vi "7.0-Convert Tabs.vi"(1 "Tab Control":T1(ring)) -> (0 "7.0 GUI Tab Equivalent State":T2)   [LabVIEW 2010]
uses:
  7.0-OCU State.ctl
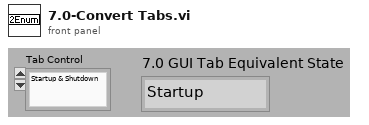
[diagram p1: front panel]
types:
  T1 = enum32{"Startup & Shutdown", "Self Test", "Manual Mode", "Auto Mode", "Mission Planning", "Timing"}
  T2 = typedef "7.0-OCU State.ctl" = enum16{"Startup", "Self Test", "Manual Mode", "Auto Mode", "Plan Mission", "Shutdown"}
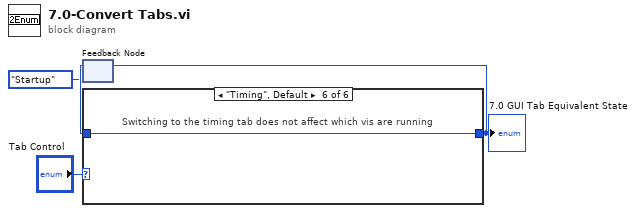
[diagram p0: block diagram]
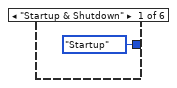
[diagram p2: hidden frame]
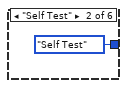
[diagram p3: hidden frame]
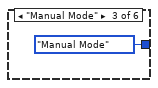
[diagram p4: hidden frame]
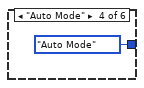
[diagram p5: hidden frame]
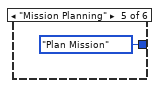
[diagram p6: hidden frame]
diagram:
  n1 = feedback #1(7.0-OCU_State."Startup" ("7.0 GUI Tab Equivalent State")) -> (w2:T2)
  n2 = case shown="\"Timing\", Default" "Tab Control" {
    tunnel: [7.0-OCU_State."Startup" ("7.0 GUI Tab Equivalent State") 7.0-OCU_State."Self Test" ("7.0 GUI Tab Equivalent State") 7.0-OCU_State."Manual Mode" ("7.0 GUI Tab Equivalent State") 7.0-OCU_State."Auto Mode" ("7.0 GUI Tab Equivalent State") 7.0-OCU_State."Plan Mission" ("7.0 GUI Tab Equivalent State") w10] -> w3
    tunnel: w2 -> [_ _ _ _ _ w10]
    frame "Startup & Shutdown" {
    }
    frame "Self Test" {
    }
    frame "Manual Mode" {
    }
    frame "Auto Mode" {
    }
    frame "Mission Planning" {
    }
    frame "Timing", Default {
      # "Switching to the timing tab does not affect which vis are running"
    }
  }
  "7.0 GUI Tab Equivalent State" <- w3
  n3 = feedback-in #1(w3) -> ()
